vi "torque transducer test.vi"() -> ()   [LabVIEW 2025]
uses:
  Classes/Torque Transducer/Torque Transducer.lvclass
panel:
  in  "Torque Transducer.lvclass":refnum<class "Torque Transducer.lvclass">
  in  "stop 2":bool
  out "error out 2":errorcluster
  out "error out":errorcluster
  out "Waveform Chart":dbl(graph)
  in  "stop":bool
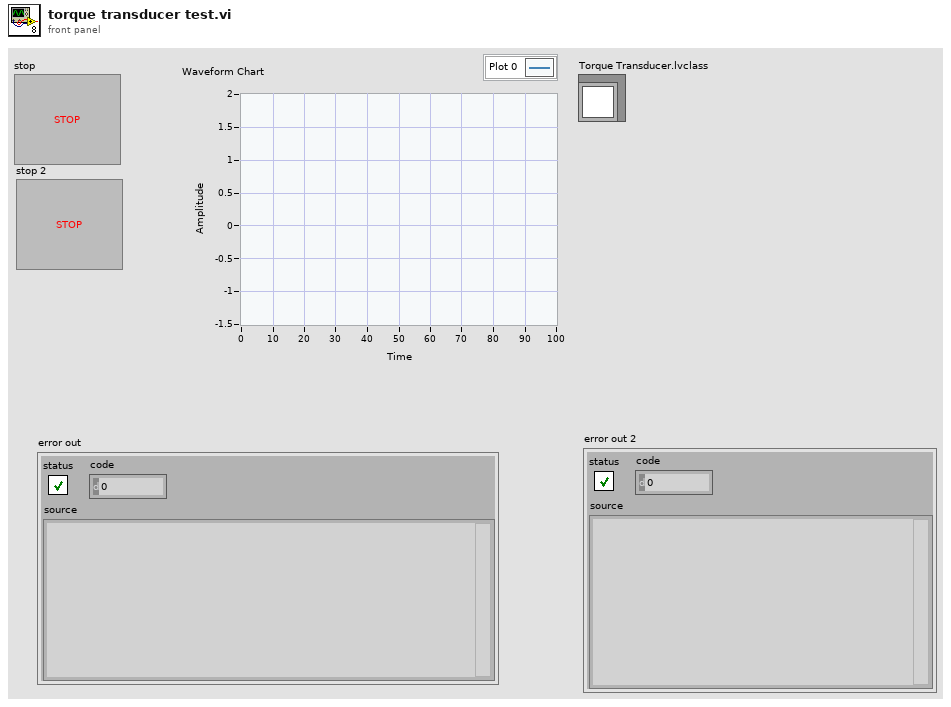
[diagram p1: front panel]
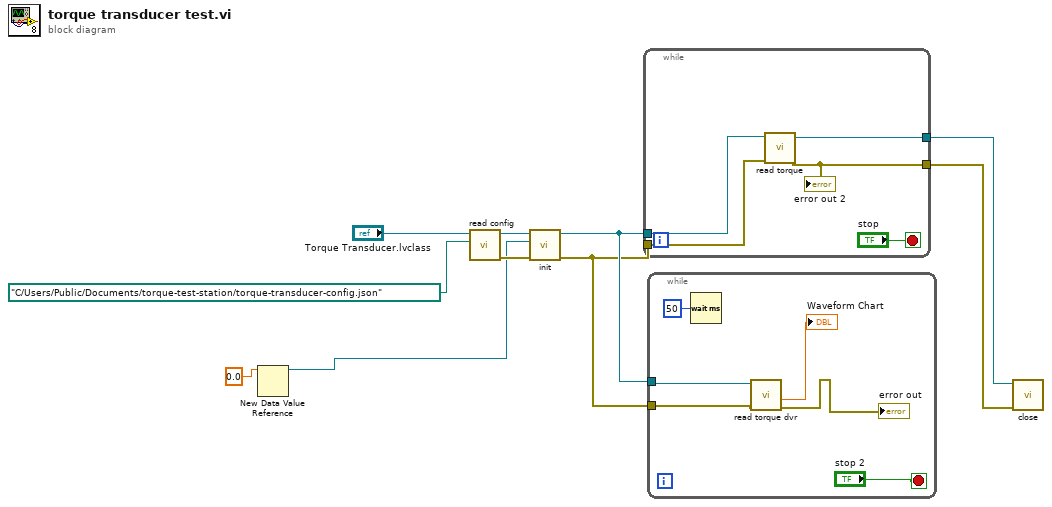
[diagram p0: block diagram]
diagram:
  n1 = New Data Value Reference(data value=0.0) -> (data value reference=w2:refnum<data-value>)  [unwired: 1 in, 1 out]
  n2 = call-dynamic "read config.vi"("Path"=path "C:/Users/Public/Documents/torque-test-station/torque-transducer-config.json", "Torque Transducer in"="Torque Transducer.lvclass") -> ("error out"=w7:errorcluster, "Torque Transducer out"=w8:refnum<class "Torque Transducer.lvclass">)  [unwired: 8 in]
  n3 = call-dynamic "init.vi"("error in (no error)"=w7, "Torque Value"=w2, "Torque Transducer in"=w8) -> ("error out"=w1:errorcluster, "Torque Transducer out"=w6:refnum<class "Torque Transducer.lvclass">)  [unwired: 7 in]
  n4 = while {
    tunnel: w6 -> [w15]
    tunnel: w1 -> [w14]
    tunnel: [w12] -> w4
    tunnel: [w11] -> w5
    stop <- "stop" stop-if-true
    n5 = call-dynamic "read torque.vi"("error in (no error)"=w14, "Torque Transducer in"=w15) -> ("error out"=w12:errorcluster, "Torque Transducer out"=w11:refnum<class "Torque Transducer.lvclass">)  [unwired: 8 in]
    "error out 2" <- w12
  }
  n6 = while {
    tunnel: w6 -> [w20]
    tunnel: w1 -> [w19]
    stop <- "stop 2" stop-if-true
    n7 = Wait (ms)(milliseconds to wait=u32 50) -> ()  [unwired: 1 out]
    n8 = call-dynamic "read torque dvr.vi"("error in (no error)"=w19, "Torque Transducer in"=w20) -> ("error out"=→"error out":errorcluster, "Torque"=→"Waveform Chart":dbl)  [unwired: 6 in, 2 out]
  }
  n9 = call-dynamic "close.vi"("error in (no error)"=w4, "Torque Transducer in"=w5) -> ()  [unwired: 8 in, 2 out]
